vi "empty_inline_shared_reentrant.vi"   [LabVIEW 2026]
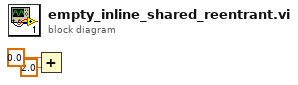
[diagram p0: block diagram]
diagram:
  n1 = Add(x=0.0, y=2.0) -> ()  [unwired: 1 out]
